vi "CRYGet Input Variables from Formula.vi"(11 "Formula string":string="X3y56y78+X27yu6t+58989;") -> (3 "Variables Out":string[](array[string]))   [LabVIEW 2013]
uses:
  <vilib>/regexp/Match Regular Expression.xnode
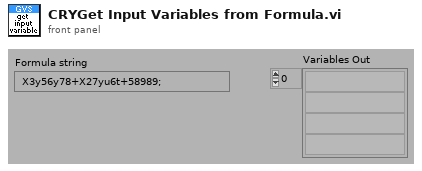
[diagram p1: front panel]
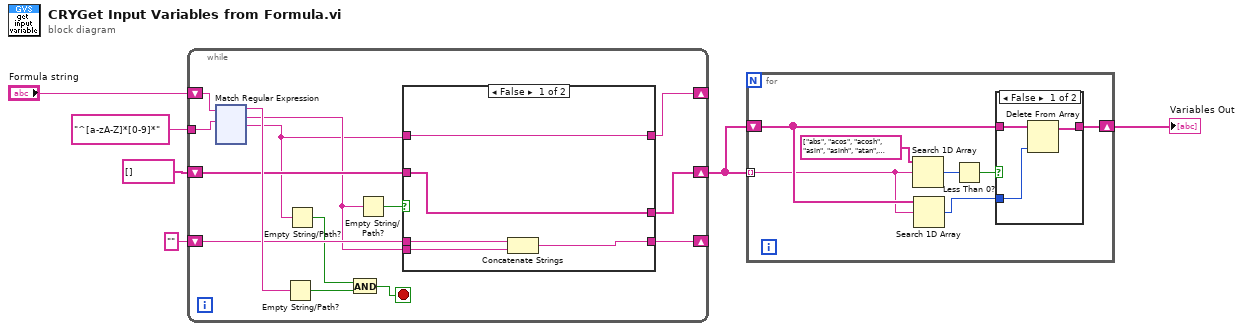
[diagram p0: block diagram]
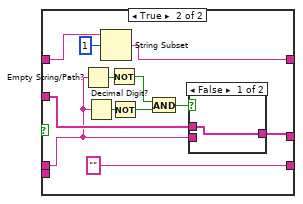
[diagram p3: hidden frame]
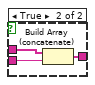
[diagram p4: hidden frame]
diagram:
  n1 = while {
    tunnel: "^[a-zA-Z]*[0-9]*" ("regular expression") -> [w17]
    shift-right: [w14] -> _
    shift-left: "Formula string" -> [w18]
    shift-right: [w12] -> w2
    shift-left: string[] [] ("Array") -> [w13]
    shift-right: [w11] -> _
    shift-left: "" ("after match") -> [w10]
    stop <- w19 stop-if-true
    n2 = xnode "Match Regular Expression"("input string"=w18, "regular expression"=w17) -> ("before match"=w16:string, "whole match"=w9:string, "after match"=w8:string)  [unwired: 4 in, 2 out]
    n3 = Empty String/Path?(string/path=w16) -> (empty?=w20:bool)
    n4 = Empty String/Path?(string/path=w8) -> (empty?=w7:bool)
    n5 = And(x=w7, y=w20) -> (x .and. y?=w19:bool)
    n6 = Empty String/Path?(string/path=w9) -> (empty?=w15:bool)
    n7 = case shown="False" w15 {
      tunnel: w8 -> [w21 w36]
      tunnel: [w21 w35] -> w14
      tunnel: w13 -> [w25 w33]
      tunnel: [w25 w32] -> w12
      tunnel: [w23 "" ("after match")] -> w11
      tunnel: w10 -> [w24 w30]
      tunnel: w9 -> [w22 _]
      frame False {
        n8 = Concatenate Strings(w24, w22) -> (w23:string)
      }
      frame True {
        n9 = Empty String/Path?(string/path=w30) -> (empty?=w31:bool)
        n10 = Decimal Digit?(1:w30) -> (0:w29:bool)
        n11 = String Subset(string=w36, offset (0)=1) -> (substring=w35:string)  [unwired: 1 in]
        n12 = Not(x=w31) -> (.not. x?=w28:bool)
        n13 = Not(x=w29) -> (.not. x?=w27:bool)
        n14 = And(x=w28, y=w27) -> (x .and. y?=w26:bool)
        n15 = case shown="False" w26 {
          tunnel: w33 -> [w38 w41]
          tunnel: [w38 w40] -> w32
          tunnel: w30 -> [_ w39]
          frame False {
          }
          frame True {
            n16 = Build Array (concatenate)(w41, w39) -> (w40:string[])
          }
        }
      }
    }
  }
  n17 = for {
    tunnel: w2 -> [w154] mode=indexing
    shift-right: [w156] -> w1
    shift-left: w2 -> [w155]
    n18 = Search 1D Array(1D array=string[] ["abs", "acos", "acosh", "asin", "asinh", "atan", "atan2", "atanh", "ceil", "cos", "cosh", "cot", "csc", "exp", "expm1", "floor", "getexp", "getman", "int", "intrz", "ln", "lnp1", "log", "log2", "max", "min", "mod", "pow", "rand", "rem", "sec", "sign", "sin", "sinc", "sinh", "sizeOfDim", "sqrt", "tan", "tanh"] ("Array"), element=w154) -> (index of element=w158:i32)  [unwired: 1 in]
    n19 = Search 1D Array(1D array=w155, element=w154) -> (index of element=w153:i32)  [unwired: 1 in]
    n20 = Less Than 0?(x=w158) -> (x < 0?=w157:bool)
    n21 = case shown="False" w157 {
      tunnel: w155 -> [w162 w163]
      tunnel: [w161 w163] -> w156
      tunnel: w153 -> [w160 _]
      frame False {
        n22 = Delete From Array(array=w162, index=w160) -> (array with subset deleted=w161:string[])  [unwired: 1 in, 1 out]
      }
      frame True {
      }
    }
  }
  "Variables Out" <- w1
